vi "chnage allchild cell.vi"(9 "Active Cell:String":string, 10 "all childtag":string[](array[string]), 11 "ChannalConfig":refnum<vi>) -> ()   [LabVIEW 2011]
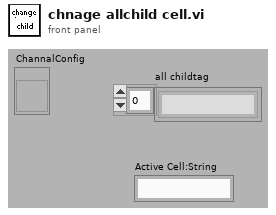
[diagram p1: front panel]
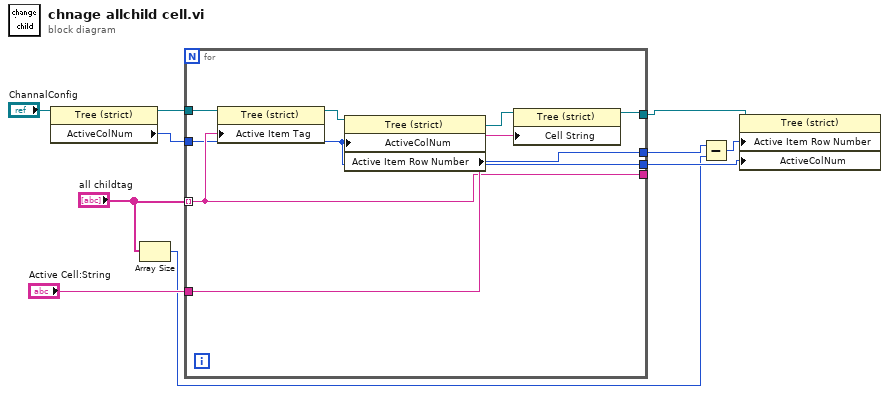
[diagram p0: block diagram]
diagram:
  n1 = property class="Tree (strict)"(reference="ChannalConfig") -> (reference out=w9:refnum<vi>, "ActiveColNum"=w8:i32)  [unwired: 1 in, 1 out]
  n2 = Array Size(array="all childtag") -> (size(s)=w2:i32)
  n3 = for {
    tunnel: w9 -> [w18]
    tunnel: w8 -> [w12]
    tunnel: "Active Cell:String" -> [w15]
    tunnel: "all childtag" -> [w13] mode=indexing
    tunnel: [w14] -> w5
    tunnel: [w13] -> _
    tunnel: [w12] -> w6
    tunnel: [w11] -> w3
    n4 = property class="Tree (strict)"(reference=w18, "Active Item Tag"=w13) -> (reference out=w17:refnum<vi>)  [unwired: 1 in, 1 out]
    n5 = property class="Tree (strict)"(reference=w17, "ActiveColNum"=w12) -> (reference out=w16:refnum<vi>, "Active Item Row Number"=w11:i32)  [unwired: 1 in, 1 out]
    n6 = property class="Tree (strict)"(reference=w16, "Cell String"=w15) -> (reference out=w14:refnum<vi>)  [unwired: 1 in, 1 out]
  }
  n7 = Subtract(x=w3, y=w2) -> (x-y=w1:i32)
  n8 = property class="Tree (strict)"(reference=w5, "Active Item Row Number"=w1, "ActiveColNum"=w6) -> ()  [unwired: 1 in, 2 out]
